vi "Read Cap to sweep.vi"(11 "Toggle 6 in":refnum<class "Toggle 6.lvclass">) -> (2 "Cap to sweep":T1[](array[typedef]), 3 "Toggle 6 out":refnum<class "Toggle 6.lvclass">)   [LabVIEW 2020, in "Toggle 6.lvclass"]
uses:
  Toggle 6.lvclass
  Controls/Parameter Cluster.ctl
  Toggle 6.lvclass/Toggle 6.ctl
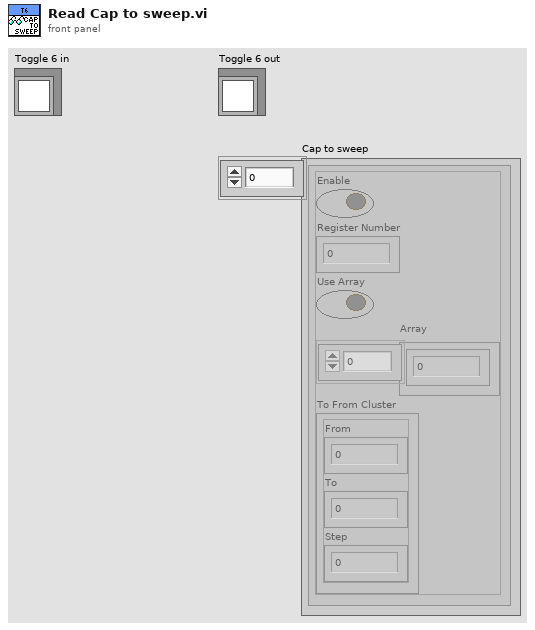
[diagram p1: front panel]
types:
  T1 = typedef "Toggle 6.lvclass/Parameter Cluster.ctl" = cluster{"Enable":bool, "Register Number":u32, "Use Array":bool, "Array":dbl[], "To From Cluster":cluster{"From":dbl, "To":dbl, "Step":dbl}}
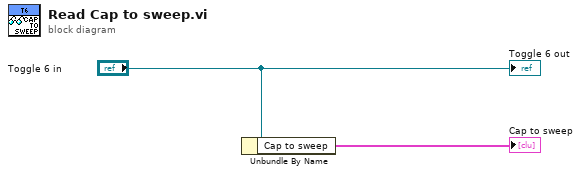
[diagram p0: block diagram]
diagram:
  n1 = Unbundle By Name("Toggle 6 in") -> ("Cap to sweep"=→"Cap to sweep":T1[])
  "Toggle 6 out" <- "Toggle 6 in"
